vi "Get Target XML Information.vi"(8 "error in":errorcluster, 11 "DOM document":refnum<k20>) -> (0 "error out":errorcluster, 2 "target xml information":T1[](array[typedef]), 3 "DOM document out":refnum<k20>)   [LabVIEW 2020, in "Template Tool.lvlib"]
uses:
  Template Tool.lvlib
  <resource>/objmgr/DOMUserDefRef.rc
  <vilib>/xml/NI_XML.lvlib
  <vilib>/xml/Close Reference(Node).vi
  Target XML Information.ctl
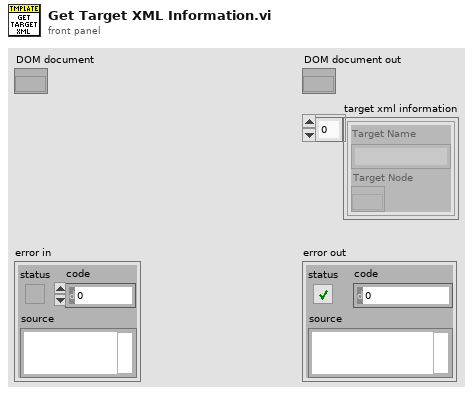
[diagram p1: front panel]
types:
  T1 = typedef "Template Tool.lvlib/Target XML Information.ctl" = cluster{"Target Name":string, "Target Node":refnum<k20>}
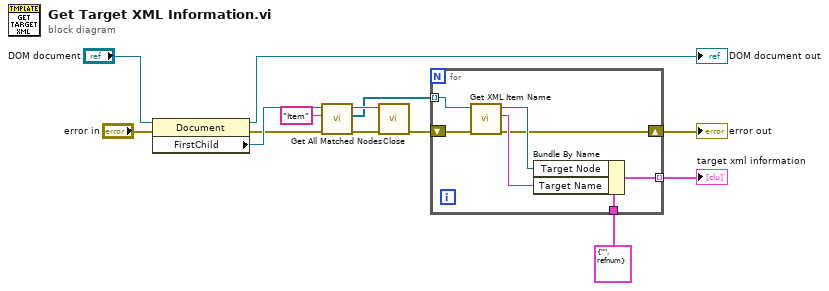
[diagram p0: block diagram]
diagram:
  n1 = property class="Document"(reference="DOM document", error in="error in") -> (reference out=→"DOM document out":refnum<k20>, error out=w11:errorcluster, "FirstChild"=w13:refnum<k20>)
  n2 = call <vilib>:"Get All Matched Nodes.vi"("error in (no error)"=w11, "XPath expression"="Item", "node in"=w13) -> ("error out"=w10:errorcluster, "node result array"=w5:refnum<k20>[], "node out"=w9:refnum<k20>)  [unwired: 6 in]
  n3 = call-poly <vilib>:"Close.vi"("error in (no error)"=w10, "node"=w9) -> ("error out"=w6:errorcluster)  [unwired: 7 in]
  n4 = for {
    shift-right: [w15] -> w3
    shift-left: w6 -> [w20]
    tunnel: w5 -> [w19] mode=indexing
    tunnel: T1 {"Target Name"="", "Target Node"=refnum} ("Target XML Info") -> [w18]
    tunnel: [w14] -> w1 mode=indexing
    n5 = call "Get XML Item Name.vi"("error in"=w20, "Node"=w19) -> ("error out"=w15:errorcluster, "Name"=w17:string, "Node out"=w16:refnum<k20>)  [unwired: 7 in]
    n6 = Bundle By Name(cluster=w18, "Target Node"=w16, "Target Name"=w17) -> (w14:T1)
  }
  "error out" <- w3
  "target xml information" <- w1
